vi "Destroy Channel.vi"(8 "error in (no error)":errorcluster, 10 "Channel Name":string, 11 "CIFCorePlugin in":refnum<class "CIFCorePlugin.lvclass">) -> (0 "error out":errorcluster, 3 "CIFCorePlugin out":refnum<class "CIFCorePlugin.lvclass">)   [LabVIEW 2021, in "CIFCorePlugin.lvclass"]
uses:
  CIFCorePlugin.lvclass
  CIFCorePlugin.lvclass/CIFCorePlugin.ctl
  CIFUtilities/CIFChannelMng/CIFChannelMng.lvclass
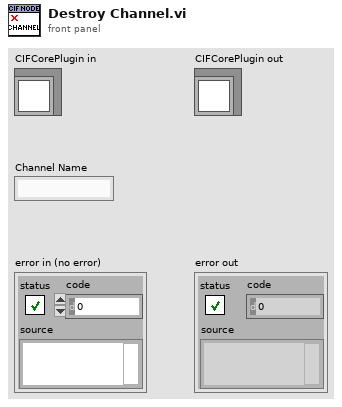
[diagram p1: front panel]
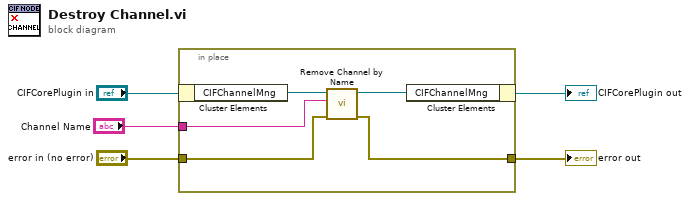
[diagram p0: block diagram]
diagram:
  n1 = in-place {
    in-place-border: "error in (no error)" -> [w8]
    in-place-border: [w7] -> w4
    in-place-border: "Channel Name" -> [w6]
    n2 = in-place-cluster #1("CIFCorePlugin in") -> ("CIFChannelMng"=w10:refnum<class "CIFChannelMng.lvclass">)
    n3 = call "Remove Channel by Name.vi"("error in (no error)"=w8, "Channel Name"=w6, "CIFChannelMng in"=w10) -> ("error out"=w7:errorcluster, "CIFChannelMng out"=w9:refnum<class "CIFChannelMng.lvclass">)  [unwired: 7 in]
    n4 = in-place-cluster #1("CIFChannelMng"=w9) -> (→"CIFCorePlugin out":refnum<class "CIFCorePlugin.lvclass">)
  }
  "error out" <- w4
